vi "ReadCustomData.vi"(8 "error in":errorcluster, 10 "Key":string, 11 "Image Reference In":T1) -> (0 "error out":errorcluster, 2 "Data":string, 3 "Image Reference Out":T1)   [LabVIEW 2024, in "OpenLvVision_Image.lvlib" / "Management.lvlib"]
doc: "Reads the data associated with a specific custom key stored within the image's data."
uses:
  Management.lvlib
  TypeDef/Image.ctl
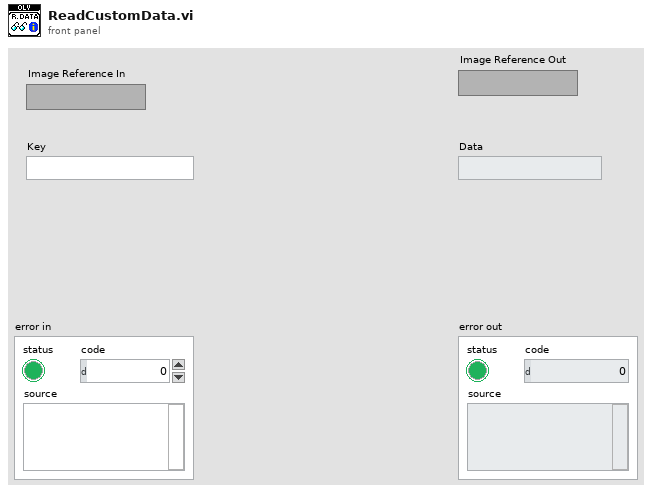
[diagram p1: front panel]
types:
  T1 = typedef "OpenLvVision_Image.lvlib/Management.lvlib/Image.ctl" = refnum<image>
  T2 = typedef "IMAQ Image.ctl" = refnum<image>
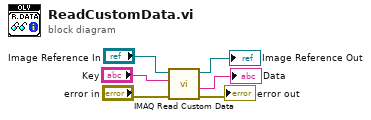
[diagram p0: block diagram]
diagram:
  n1 = call "IMAQ Read Custom Data"("error in (no error)"="error in", "Key"="Key", "Image"="Image Reference In") -> ("error out"=→"error out":errorcluster, "Custom Data Out"=→"Data":string, "Image (duplicate)"=→"Image Reference Out":T2)  [unwired: 6 in]
